vi "GlobalPath.vi"() -> ()   [LabVIEW 2015]
panel:
  in  "AthinaOutDataDir":path=path "/home/atlas/Micromegas/M0Data"
  in  "DBpath":path=path "/home/atlas/Micromegas/M0Data/dbtxtfiles"
  in  "RootMacroDir":path=path "/home/atlas/Micromegas/root_macro"
  in  "ViDir":path=path "/home/atlas/Micromegas/interface"
  in  "OutDataDir":path=path "/home/atlas/Micromegas/M0Data"
  in  "LogFilesDir":path=path "/home/atlas/Micromegas/M0Data/logfiles"
  in  "BinDir":path=path "/home/atlas/Micromegas/bin"
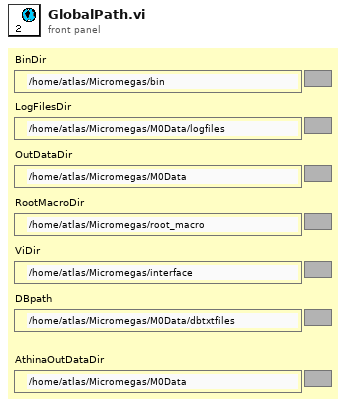
[diagram p1: front panel]
diagram:
